vi "Get Laptop Power Remaning.vi"() -> (3 "BatteryLifePercent":u8)   [LabVIEW 2023]
uses:
  <vilib>/Rock Robotics/Network Tables/NT Write Integer.vi
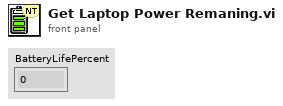
[diagram p1: front panel]
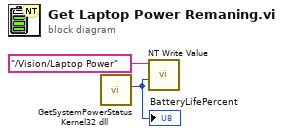
[diagram p0: block diagram]
diagram:
  n1 = call "GetSystemPowerStatus Kernel32 dll.vi"() -> ("BatteryLifePercent"=w1:u8)  [unwired: 11 in]
  "BatteryLifePercent" <- w1
  n2 = call-poly <vilib>:"NT Write Value.vi"("value"=w1, "name"="/Vision/Laptop Power" ("Name")) -> ()  [unwired: 9 in, 1 out]
